vi "Overlay PAResults.vi"(6 "Color":u32[](array[colorbox])=[6618880, 16860, 16774930, 3381759, 9567230], 7 "Group":string, 8 "error in":errorcluster, 9 "Overlay Type":u16[](array[ring]) items=["Rectangle", "Numbers", "Points", "Lines(Start,End)"], 10 "Particle Measurements (Pixels)":dbl[][](array[numeric]) format="%.2f", 11 "Image":T1) -> (0 "error out":errorcluster, 3 "Image Out":T1)   [LabVIEW 2016]
doc: "Overlay targets at the location of the feature points in the specified colors."
uses:
  <vilib>/vision/Image Controls.llb/IMAQ Image.ctl
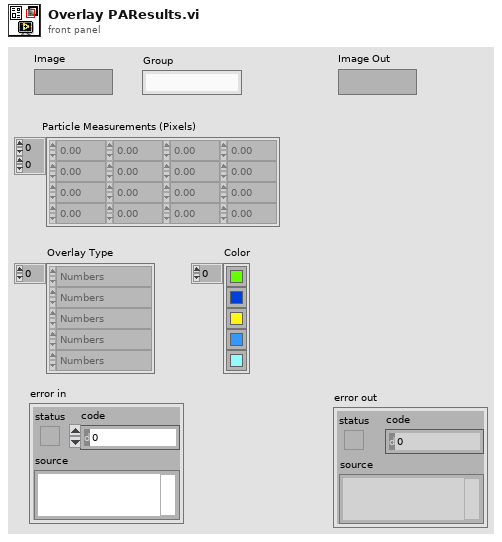
[diagram p1: front panel]
types:
  T1 = typedef "IMAQ Image.ctl" = refnum<image>
  T2 = cluster{"Numeric":i32, "Numeric":i32, "Numeric":i32, "Numeric":i32}
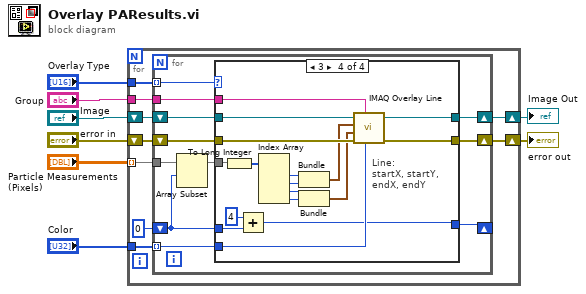
[diagram p0: block diagram]
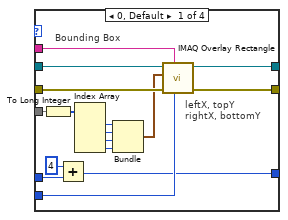
[diagram p2: hidden frame]
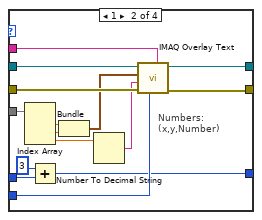
[diagram p3: hidden frame]
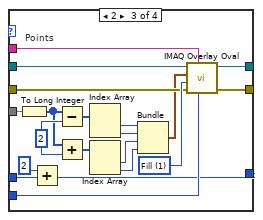
[diagram p4: hidden frame]
diagram:
  n1 = for {
    tunnel: "Color" -> [w16]
    tunnel: "Group" -> [w13]
    tunnel: "Particle Measurements (Pixels)" -> [w11] mode=indexing
    tunnel: "Overlay Type" -> [w10]
    shift-right: [w17] -> w8
    shift-left: "Image" -> [w15]
    shift-right: [w12] -> w4
    shift-left: "error in" -> [w14]
    n2 = for {
      tunnel: w10 -> [w27] mode=indexing
      tunnel: w11 -> [w20]
      tunnel: w13 -> [w26]
      tunnel: w16 -> [w23] mode=indexing
      shift-right: [w22] -> w17
      shift-left: w15 -> [w28]
      shift-right: [w24] -> w12
      shift-left: w14 -> [w25]
      shift-right: [w21] -> _
      shift-left: 0 -> [w19]
      n3 = Array Subset(array=w20, index=w19) -> (w18:dbl[])  [unwired: 1 in]
      n4 = case shown="3" w27 {
        tunnel: w28 -> [w44 w57 w77 w96]
        tunnel: w18 -> [w30 w45 w69 w81]
        tunnel: w26 -> [w43 w59 w72 w95]
        tunnel: w25 -> [w42 w58 w76 w94]
        tunnel: [w41 w55 w74 w93] -> w24
        tunnel: w23 -> [w40 w53 w71 w92]
        tunnel: [w39 w54 w73 w91] -> w22
        tunnel: w19 -> [w33 w48 w61 w83]
        tunnel: [w31 w46 w60 w82] -> w21
        frame 0, Default {
          # "Bounding Box"
          # "leftX, topY\nrightX, bottomY"
          n5 = To Long Integer(number=w30) -> (32bit integer=w29:i32[])
          n6 = Add(x=4 ("length"), y=w33) -> (x+y=w31:i32)
          n7 = Index Array(array=w29) -> (element #1=w38:i32, element #2=w37:i32, element #3=w36:i32, element #4=w35:i32)  [unwired: 4 in]
          n8 = Bundle("Numeric"=w38, "Numeric"=w37, "Numeric"=w36, "Numeric"=w35) -> (w34:T2)  [unwired: 1 in]
          n9 = call "IMAQ Overlay Rectangle"("Color"=w40, "Group"=w43, "error in (no error)"=w42, "Rectangle"=w34, "Image"=w44) -> ("error out"=w41:errorcluster, "Image Out"=w39:T1)  [unwired: 5 in]
        }
        frame 1 {
          # "Numbers:\n(x,y,Number)"
          n10 = Index Array(array=w45) -> (element #1=w52:dbl, element #2=w51:dbl, element #3=w49:dbl)  [unwired: 3 in]
          n11 = Add(x=3, y=w48) -> (x+y=w46:i32)
          n12 = Bundle("Numeric"=w52, "Numeric"=w51) -> (w50:cluster{"Numeric":dbl, "Numeric":dbl})  [unwired: 1 in]
          n13 = Number To Decimal String(number=w49) -> (decimal integer string=w56:string)  [unwired: 1 in]
          n14 = call "IMAQ Overlay Text"("Group"=w59, "Text Color (black)"=w53, "error in (no error)"=w58, "String"=w56, "Origin"=w50, "Image"=w57) -> ("error out"=w55:errorcluster, "Image Out"=w54:T1)  [unwired: 4 in]
        }
        frame 2 {
          w79 = u32 1 items=["Frame", "Fill"] ("Drawing Mode (Frame)")
          w78 = 2
          # "Points"
          n15 = To Long Integer(number=w69) -> (32bit integer=w70:i32[])
          n16 = Add(x=2, y=w61) -> (x+y=w60:i32)
          n17 = Subtract(x=w70, y=w78) -> (x-y=w68:i32[])
          n18 = Add(x=w70, y=w78) -> (x+y=w67:i32[])
          n19 = Index Array(array=w68) -> (element #1=w66:i32, element #2=w65:i32)  [unwired: 2 in]
          n20 = Index Array(array=w67) -> (element #1=w64:i32, element #2=w63:i32)  [unwired: 2 in]
          n21 = Bundle(w66, w65, w64, w63) -> (w75:cluster{i32, i32, i32, i32})  [unwired: 1 in]
          n22 = call "IMAQ Overlay Oval"("Color"=w71, "Group"=w72, "error in (no error)"=w76, "Drawing Mode (Frame)"=w79, "Bounding Rectangle"=w75, "Image"=w77) -> ("error out"=w74:errorcluster, "Image Out"=w73:T1)  [unwired: 4 in]
        }
        frame 3 {
          # "Line:\nstartX, startY, endX, endY"
          n23 = To Long Integer(number=w81) -> (32bit integer=w80:i32[])
          n24 = Add(x=4 ("length"), y=w83) -> (x+y=w82:i32)
          n25 = Index Array(array=w80) -> (element #1=w90:i32, element #2=w89:i32, element #3=w88:i32, element #4=w87:i32)  [unwired: 4 in]
          n26 = Bundle("Numeric"=w90, "Numeric"=w89) -> (w86:cluster{"Numeric":i32, "Numeric":i32})  [unwired: 1 in]
          n27 = Bundle("Numeric"=w88, "Numeric"=w87) -> (w85:cluster{"Numeric":i32, "Numeric":i32})  [unwired: 1 in]
          n28 = call "IMAQ Overlay Line"("Color"=w92, "Group"=w95, "error in (no error)"=w94, "End Point"=w85, "Start Point"=w86, "Image"=w96) -> ("error out"=w93:errorcluster, "Image Out"=w91:T1)  [unwired: 4 in]
        }
      }
    }
  }
  "Image Out" <- w8
  "error out" <- w4
